vi "Write Thermocouple Type.vi"(8 "error in":errorcluster, 10 "thermocouple type":T1, 11 "thermocouple channel in":refnum<class "Thermocouple Channel.lvclass">) -> (0 "error out":errorcluster, 3 "thermocouple channel out":refnum<class "Thermocouple Channel.lvclass">)   [LabVIEW 2020, in "Scan Engine Scripting.lvlib" / "Thermocouple Channel.lvclass"]
uses:
  Thermocouple Channel.lvclass
  Thermocouple Type.ctl
  Thermocouple Channel.lvclass/Thermocouple Channel.ctl
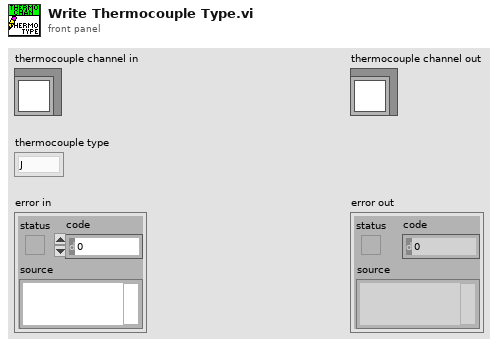
[diagram p1: front panel]
types:
  T1 = typedef "Scan Engine Scripting.lvlib/Thermocouple Channel.lvclass/Thermocouple Type.ctl" = enum16{"J", "K", "T", "E", "R", "S", "N", "B"}
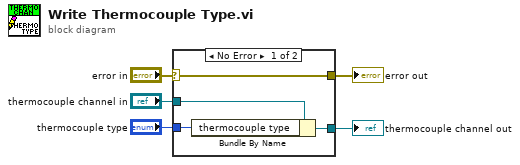
[diagram p0: block diagram]
diagram:
  n1 = case shown="No Error" "error in" {
    selector: "error in" -> [w9 w10]
    tunnel: [w9 w10] -> w4
    tunnel: [w7 w11] -> w2
    tunnel: "thermocouple channel in" -> [w8 w11]
    tunnel: "thermocouple type" -> [w6 _]
    frame No Error {
      n2 = Bundle By Name(cluster=w8, "thermocouple type"=w6) -> (w7:refnum<class "Thermocouple Channel.lvclass">)
    }
    frame Error {
    }
  }
  "error out" <- w4
  "thermocouple channel out" <- w2
